vi "WaitForMove.vi"(8 "error in (no error)":errorcluster, 11 "Tapedrive Object":refnum<class "Tapedrive_ESP301.lvclass">) -> (0 "error out (no error)":errorcluster, 2 "new commands":string, 3 "Tapedrive Object 2":refnum<class "Tapedrive_ESP301.lvclass">)   [LabVIEW 2013, in "Tapedrive_ESP301.lvclass"]
uses:
  Tapedrive_ESP301.lvclass
panel:
  out "Boolean":bool
  out "Position (units) 2":dbl format="%.6g"
  out "targetpos":dbl
  out "Position (units)":dbl(graph)
  out "Waveform Graph 2":dbl[][](graph)
  out "Waveform Graph":dbl[](graph)
  out "Numeric":i32
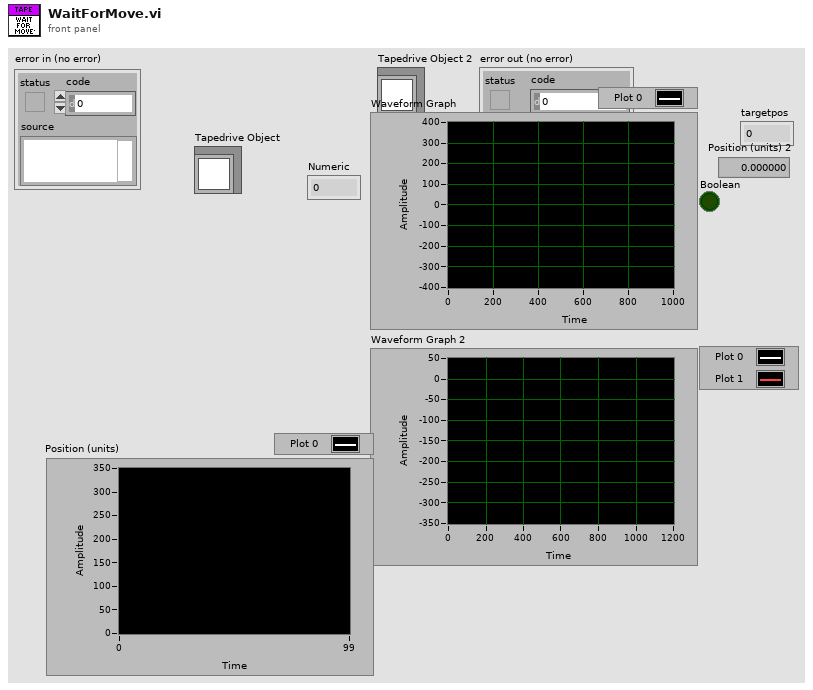
[diagram p1: front panel]
types:
  T1 = typedef "Direction.ctl" = enum16{"Forward", "Backward", "Undefined"}
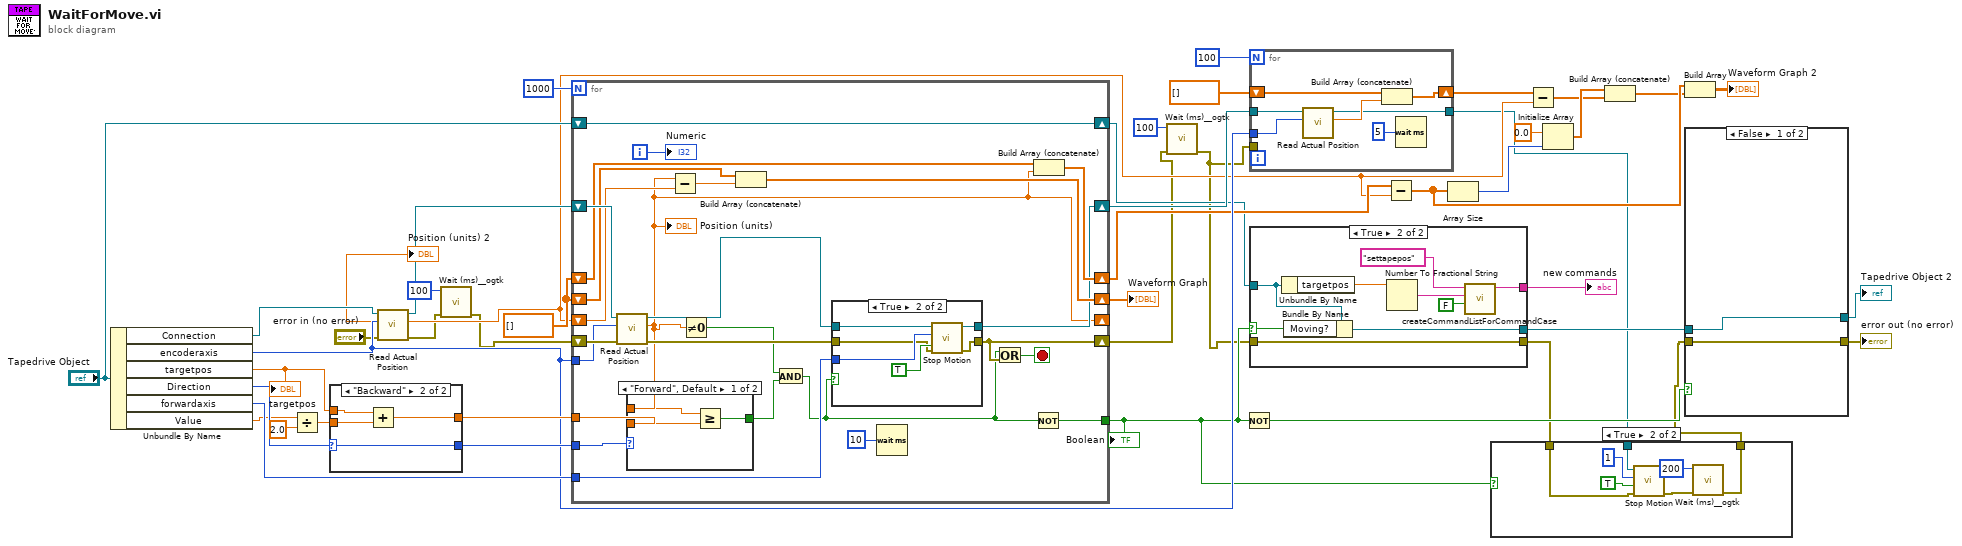
[diagram p0: block diagram]
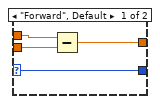
[diagram p4: hidden frame]
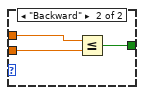
[diagram p7: hidden frame]
diagram:
  w35 = dbl[] []
  n1 = Unbundle By Name("Tapedrive Object") -> ("Connection"=w38:refnum<visa-resource-name>, "encoderaxis"=w32:i16, "targetpos"=w42:dbl, "Direction"=w43:T1, "forwardaxis"=w39:i16, "Value"=w30:dbl)
  "targetpos" <- w42
  n2 = Divide(x=w30, y=2.0) -> (x/y=w28:dbl)
  n3 = case shown="\"Backward\"" w43 {
    selector: w43 -> [w49 w53]
    tunnel: w42 -> [w48 w52]
    tunnel: [w49 w53] -> w41
    tunnel: w28 -> [w47 w51]
    tunnel: [w46 w50] -> w40
    frame "Forward", Default {
      n4 = Subtract(x=w48, y=w47) -> (x-y=w46:dbl)
    }
    frame "Backward" {
      n5 = Add(x=w52, y=w51) -> (x+y=w50:dbl)
    }
  }
  n6 = call <instrlib>:"Read Actual Position.vi"("error in (no error)"="error in (no error)", "Axis (1)"=w32, "VISA resource name"=w38) -> ("error out"=w6:errorcluster, "Position (units)"=w26:dbl, "VISA resource name out"=w37:refnum<visa-resource-name>)  [unwired: 2 in]
  "Position (units) 2" <- w26
  n7 = call <userlib>:"Wait (ms)__ogtk.vi"("error in (no error)"=w6, "milliseconds to wait"=u32 100) -> ("error out"=w5:errorcluster)  [unwired: 8 in, 1 out]
  n8 = for {
    N: 1000 -> [_]
    shift-right: [w75] -> w17
    shift-left: "Tapedrive Object" -> [w75]
    tunnel: w32 -> [w60]
    shift-right: [w68] -> w3
    shift-left: w5 -> [w76]
    tunnel: [w72] -> w7
    tunnel: w41 -> [w71]
    tunnel: w40 -> [w70]
    tunnel: w39 -> [w69]
    shift-right: [w57] -> _
    shift-left: w26 -> [w67]
    shift-right: [w65] -> w36
    shift-left: w35 -> [w64]
    shift-right: [w62] -> w27
    shift-left: w35 -> [w63]
    shift-right: [w61] -> w33
    shift-left: w37 -> [w77]
    i -> [w73]
    stop <- w78 stop-if-true
    n9 = call <instrlib>:"Read Actual Position.vi"("error in (no error)"=w76, "Axis (1)"=w60, "VISA resource name"=w77) -> ("error out"=w59:errorcluster, "Position (units)"=w57:dbl, "VISA resource name out"=w58:refnum<visa-resource-name>)  [unwired: 2 in]
    "Position (units)" <- w57
    n10 = case shown="\"Forward\", Default" w71 {
      tunnel: w70 -> [w88 w91]
      tunnel: w57 -> [w89 w92]
      tunnel: [w87 w90] -> w56
      frame "Forward", Default {
        n11 = Greater Or Equal?(x=w89, y=w88) -> (x >= y?=w87:bool)
      }
      frame "Backward" {
        n12 = Less Or Equal?(x=w92, y=w91) -> (x <= y?=w90:bool)
      }
    }
    n13 = Subtract(x=w57, y=w67) -> (x-y=w66:dbl)
    n14 = Not Equal To 0?(x=w57) -> (x != 0?=w55:bool)
    n15 = Build Array (concatenate)(w64, w66) -> (w65:dbl[])
    n16 = And(x=w55, y=w56) -> (x .and. y?=w54:bool)
    n17 = case shown="True" w54 {
      tunnel: w58 -> [w79 w86]
      tunnel: w69 -> [_ w85]
      tunnel: w59 -> [w80 w83]
      tunnel: [w80 w82] -> w68
      tunnel: [w79 w81] -> w61
      frame False {
      }
      frame True {
        n18 = call <instrlib>:"Stop Motion.vi"("error in (no error)"=w83, "Stop all axes (F)"=TRUE, "Axis (1)"=w85, "VISA resource name"=w86) -> ("error out"=w82:errorcluster, "VISA resource name out"=w81:refnum<visa-resource-name>)  [unwired: 2 in]
      }
    }
    n19 = Wait (ms)(milliseconds to wait=u32 10) -> ()  [unwired: 1 out]
    n20 = Or(x=w54, y=w68) -> (x .or. y?=w78:bool)
    n21 = Not(x=w54) -> (.not. x?=w72:bool)
    n22 = Build Array (concatenate)(w63, w57) -> (w62:dbl[])
    "Numeric" <- w73
  }
  "Waveform Graph" <- w36
  "Boolean" <- w7
  n23 = call <userlib>:"Wait (ms)__ogtk.vi"("error in (no error)"=w3, "milliseconds to wait"=u32 100) -> ("error out"=w1:errorcluster)  [unwired: 8 in, 1 out]
  n24 = Not(x=w7) -> (.not. x?=w14:bool)
  n25 = for {
    N: 100 -> [_]
    tunnel: w33 -> [w98]
    tunnel: w32 -> [w97]
    shift-right: [w95] -> w31
    shift-left: dbl[] [] -> [w94]
    tunnel: [w93] -> w10
    tunnel: w1 -> [_]
    n26 = call <instrlib>:"Read Actual Position.vi"("Axis (1)"=w97, "VISA resource name"=w98) -> ("Position (units)"=w96:dbl, "VISA resource name out"=w93:refnum<visa-resource-name>)  [unwired: 3 in, 1 out]
    n27 = Build Array (concatenate)(w94, w96) -> (w95:dbl[])
    n28 = Wait (ms)(milliseconds to wait=u32 5) -> ()  [unwired: 1 out]
  }
  n29 = case shown="True" w7 {
    selector: w7 -> [_ w104]
    tunnel: w1 -> [w101 w110]
    tunnel: [w101 w110] -> w9
    tunnel: [w100 w103] -> w18
    tunnel: w17 -> [w100 w105]
    tunnel: [_ w102] -> w12
    frame False {
    }
    frame True {
      n30 = Unbundle By Name(w105) -> ("targetpos"=w107:dbl)
      n31 = Bundle By Name(cluster=w105, "Moving?"=w104) -> (w103:refnum<class "Tapedrive_ESP301.lvclass">)
      n32 = Number To Fractional String(number=w107) -> (F-format string=w106:string)  [unwired: 3 in]
      n33 = call "createCommandListForCommandCase.vi"("immediate Check (only once)"=FALSE, "setvalue"=w106, "command"="settapepos") -> ("new commands"=w102:string)  [unwired: 8 in]
    }
  }
  "new commands" <- w12
  n34 = Subtract(x=w27, y=w26) -> (x-y=w24:dbl[])
  n35 = Array Size(array=w24) -> (size(s)=w23:i32)
  n36 = case shown="True" w7 {
    tunnel: w10 -> [_ w116]
    tunnel: w9 -> [w111 w115]
    tunnel: [w111 w113] -> w8
    frame False {
    }
    frame True {
      n37 = call <instrlib>:"Stop Motion.vi"("error in (no error)"=w115, "Stop all axes (F)"=TRUE, "Axis (1)"=1, "VISA resource name"=w116) -> ("error out"=w114:errorcluster)  [unwired: 2 in, 1 out]
      n38 = call <userlib>:"Wait (ms)__ogtk.vi"("error in (no error)"=w114, "milliseconds to wait"=u32 200) -> ("error out"=w113:errorcluster)  [unwired: 8 in, 1 out]
    }
  }
  n39 = Subtract(x=w31, y=w26) -> (x-y=w20:dbl[])
  n40 = Initialize Array(0.0 ("element"), w23) -> (w21:dbl[])
  n41 = Build Array (concatenate)(w21, w20) -> (w19:dbl[])
  n42 = Build Array(w24, w19) -> (→"Waveform Graph 2":dbl[][])
  n43 = case shown="False" w14 {
    tunnel: w18 -> [w120 w122]
    tunnel: w8 -> [w119 w121]
    tunnel: [w119 w121] -> w13
    tunnel: [w120 w122] -> w16
    frame False {
    }
    frame True {
    }
  }
  "Tapedrive Object 2" <- w16
  "error out (no error)" <- w13
